vi "processData.vi"(8 "error in (no error)":errorcluster, 10 "model":refnum<class "Model.lvclass">, 11 "EndingCycleState in":refnum<class "EndingCycleState.lvclass">) -> (0 "error out":errorcluster, 2 "model 2":refnum<class "Model.lvclass">, 3 "EndingCycleState out":refnum<class "EndingCycleState.lvclass">)   [LabVIEW 2013, in "EndingCycleState.lvclass"]
uses:
  EndingCycleState.lvclass
  Model/Model/Model.lvclass
  Typedefs/StateSelector.ctl
  Typedefs/M2AADTTypedefs.lvlib
  AutomatedMotionState/AutomatedMotionState.lvclass
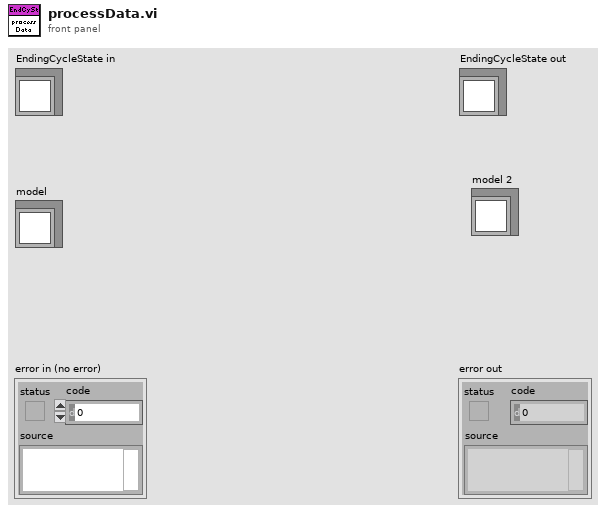
[diagram p1: front panel]
types:
  T1 = typedef "M2AADTTypedefs.lvlib/StateSelector.ctl" = enum16{"EndingCycleState", "FaultState", "InteractiveMotionState", "MovingToNewForceState", "OffState", "PausingState", "StandbyState", "StoppedState"}
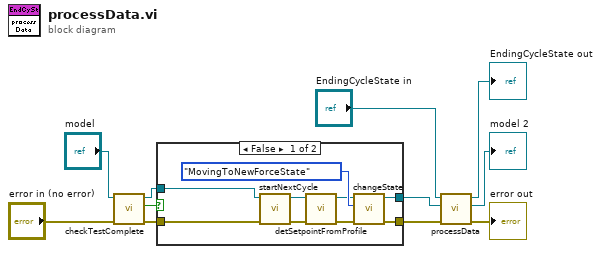
[diagram p0: block diagram]
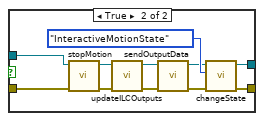
[diagram p2: hidden frame]
diagram:
  n1 = call "checkTestComplete.vi"("error in (no error)"="error in (no error)", "Model in"="model") -> ("error out"=w4:errorcluster, "testCompleteIsTrue"=w1:bool, "Model out"=w6:refnum<class "Model.lvclass">)  [unwired: 7 in]
  n2 = case shown="False" w1 {
    tunnel: w6 -> [w20 w31]
    tunnel: w4 -> [w18 w29]
    tunnel: [w17 w28] -> w3
    tunnel: [w19 w27] -> w2
    frame False {
      n3 = call "startNextCycle.vi"("error in (no error)"=w18, "Model in"=w20) -> ("error out"=w13:errorcluster, "Model out"=w15:refnum<class "Model.lvclass">)  [unwired: 8 in]
      n4 = call "detSetpointFromProfile.vi"("error in (no error)"=w13, "Model in"=w15) -> ("error out"=w12:errorcluster, "Model out"=w14:refnum<class "Model.lvclass">)  [unwired: 8 in]
      n5 = call "changeState.vi"("error in (no error)"=w12, "State:"=StateSelector."MovingToNewForceState", "Model in"=w14) -> ("error out"=w17:errorcluster, "Model out"=w19:refnum<class "Model.lvclass">)  [unwired: 7 in]
    }
    frame True {
      n6 = call "stopMotion.vi"("error in (no error)"=w29, "Model in"=w31) -> ("error out"=w22:errorcluster, "Model out"=w24:refnum<class "Model.lvclass">)  [unwired: 8 in]
      n7 = call "updateILCOutputs.vi"("error in (no error)"=w22, "Model in"=w24) -> ("error out"=w21:errorcluster, "Model out"=w23:refnum<class "Model.lvclass">)  [unwired: 8 in]
      n8 = call "sendOutputData.vi"("error in (no error)"=w21, "Model in"=w23) -> ("error out"=w26:errorcluster, "Model out"=w25:refnum<class "Model.lvclass">)  [unwired: 8 in]
      n9 = call "changeState.vi"("error in (no error)"=w26, "State:"=StateSelector."InteractiveMotionState", "Model in"=w25) -> ("error out"=w28:errorcluster, "Model out"=w27:refnum<class "Model.lvclass">)  [unwired: 7 in]
    }
  }
  n10 = call-parent "processData.vi"("error in (no error)"=w3, "model"=w2, "ControlledMotionState in"="EndingCycleState in") -> ("error out"=→"error out":errorcluster, "model 2"=→"model 2":refnum<class "Model.lvclass">, "ControlledMotionState out"=→"EndingCycleState out":refnum<class "EndingCycleState.lvclass">)  [unwired: 6 in]
